vi "set_deviceIDs.vi"(8 "error in (no error)":errorcluster caption="错误输入（无错误）", 10 "设备站点":u32[](array[numeric]), 11 "MotorSystem输入":refnum<class "MotorSystem.lvclass">) -> (0 "error out":errorcluster caption="错误输出", 3 "MotorSystem输出":refnum<class "MotorSystem.lvclass">)   [LabVIEW 2014, in "MotorSystem.lvclass"]
uses:
  MotorSystem.lvclass
  MotorSystem.lvclass/MotorSystem.ctl
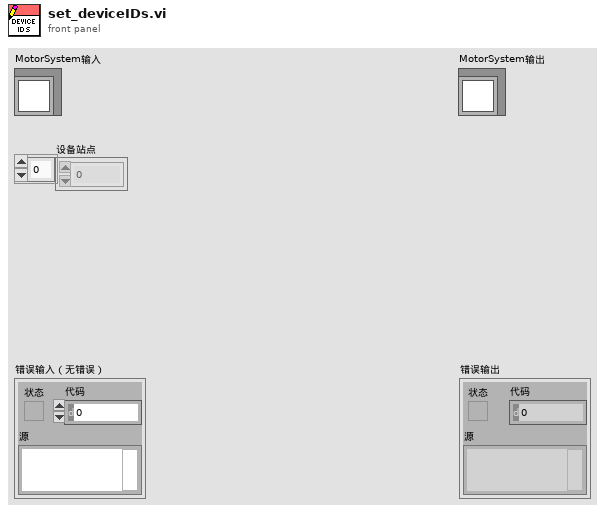
[diagram p1: front panel]
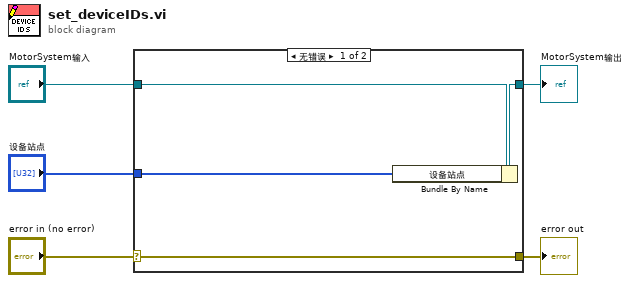
[diagram p0: block diagram]
diagram:
  n1 = case shown="无错误" "error in (no error)" {
    selector: "error in (no error)" -> [w9 w10]
    tunnel: [w9 w10] -> w4
    tunnel: [w7 w11] -> w2
    tunnel: "MotorSystem输入" -> [w8 w11]
    tunnel: "设备站点" -> [w6 _]
    frame No Error {
      n2 = Bundle By Name(cluster=w8, "设备站点"=w6) -> (w7:refnum<class "MotorSystem.lvclass">)
    }
    frame Error {
    }
  }
  "error out" <- w4
  "MotorSystem输出" <- w2
